vi "Test Array of Clusters to VMap.vi"(8 "error in":errorcluster) -> (0 "error out":errorcluster, 2 "passed":bool)   [LabVIEW 2020, in "test_openg_variant.lvlib"]
uses:
  test_openg_variant.lvlib
  <vilib>/addons/_JKI Toolkits/Caraya/classes/Test/Test.lvclass
  source/library/openg_variant.lvlib
  <vilib>/addons/_JKI Toolkits/Caraya/classes/Assert/Assert.lvclass
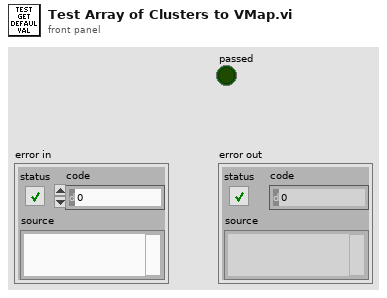
[diagram p1: front panel]
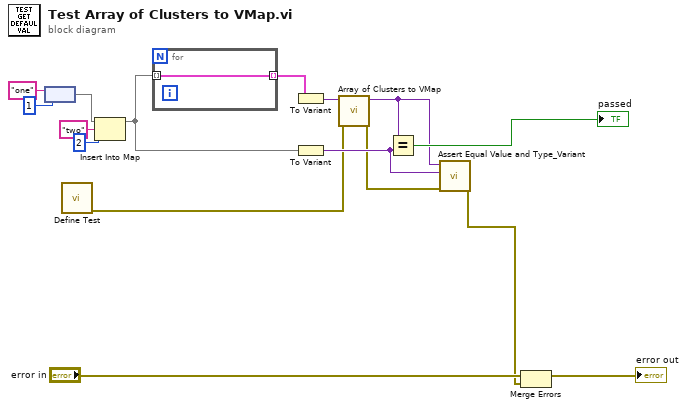
[diagram p0: block diagram]
diagram:
  n1 = node("one" ("key"), 1 ("value")) -> (w15:map{string, i32})
  n2 = call <vilib>:"Define Test.vi"() -> ("error out"=w4:errorcluster)  [unwired: 10 in, 1 out]
  n3 = Insert Into Map(map in=w15, key="two", value=2) -> (map out=w8:map{string, i32})  [unwired: 2 out]
  n4 = for {
    tunnel: w8 -> [w17] mode=indexing
    tunnel: [w17] -> w10 mode=indexing
  }
  n5 = To Variant(anything=w10) -> (Variant=w9:variant)
  n6 = To Variant(anything=w8) -> (Variant=w5:variant)
  n7 = call "Array of Clusters to VMap.vi"("error in"=w4, "Array of Clusters (key-value)"=w9) -> ("error out"=w3:errorcluster, "Map"=w6:variant)  [unwired: 8 in]
  n8 = Equal?(x=w6, y=w5) -> (x = y?=→"passed":bool)
  n9 = call <vilib>:"Assert Equal Value and Type_Variant.vi"("error in (no error)"=w3, "Y"=w5, "X"=w6) -> ("error out"=w1:errorcluster)  [unwired: 7 in, 1 out]
  n10 = Merge Errors("error in", w1) -> (→"error out":errorcluster)
